vi "LEDC Control Loop 1931 Main.vi"(0 "LEDAD Port":refnum<visa-resource-name>="COM9", 1 "Enable":u8, 2 "Inten Desired":refnum<vi>, 3 "Illum Meas":refnum<vi>, 5 "Light Meter Port":refnum<visa-resource-name>="COM3", 7 "Illum Desired":dbl, 9 "Error Margin":dbl=2.0, 11 "error in (no error)":errorcluster, 12 "Illum Cal Factor":dbl=0.444212 format="%#.6f", 13 "Stop":bool) -> (4 "LEDAD Port out":refnum<visa-resource-name>, 6 "Light Meter Port out":refnum<visa-resource-name>, 8 "Illum Meas":dbl format="%#_4g", 10 "Inten Desired":dbl, 14 "Done":bool, 15 "error out":errorcluster)   [LabVIEW 2010]
panel:
  out "Flag2":bool
  out "Flag1":bool
  out "Slope":dbl format="%#_4g"
  in  "Illum 10":dbl format="%#_4g"
  out "In Progress":bool
  in  "Illum 90":dbl format="%#_4g"
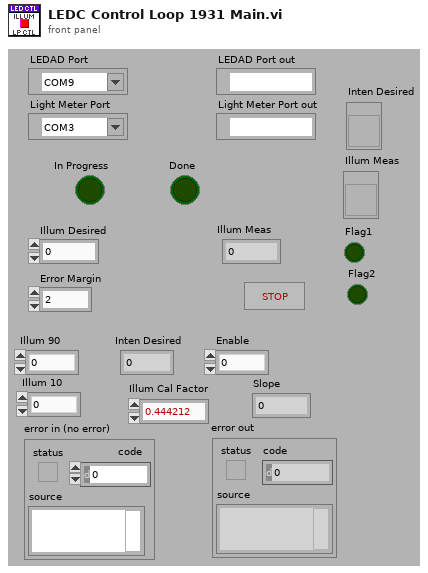
[diagram p1: front panel]
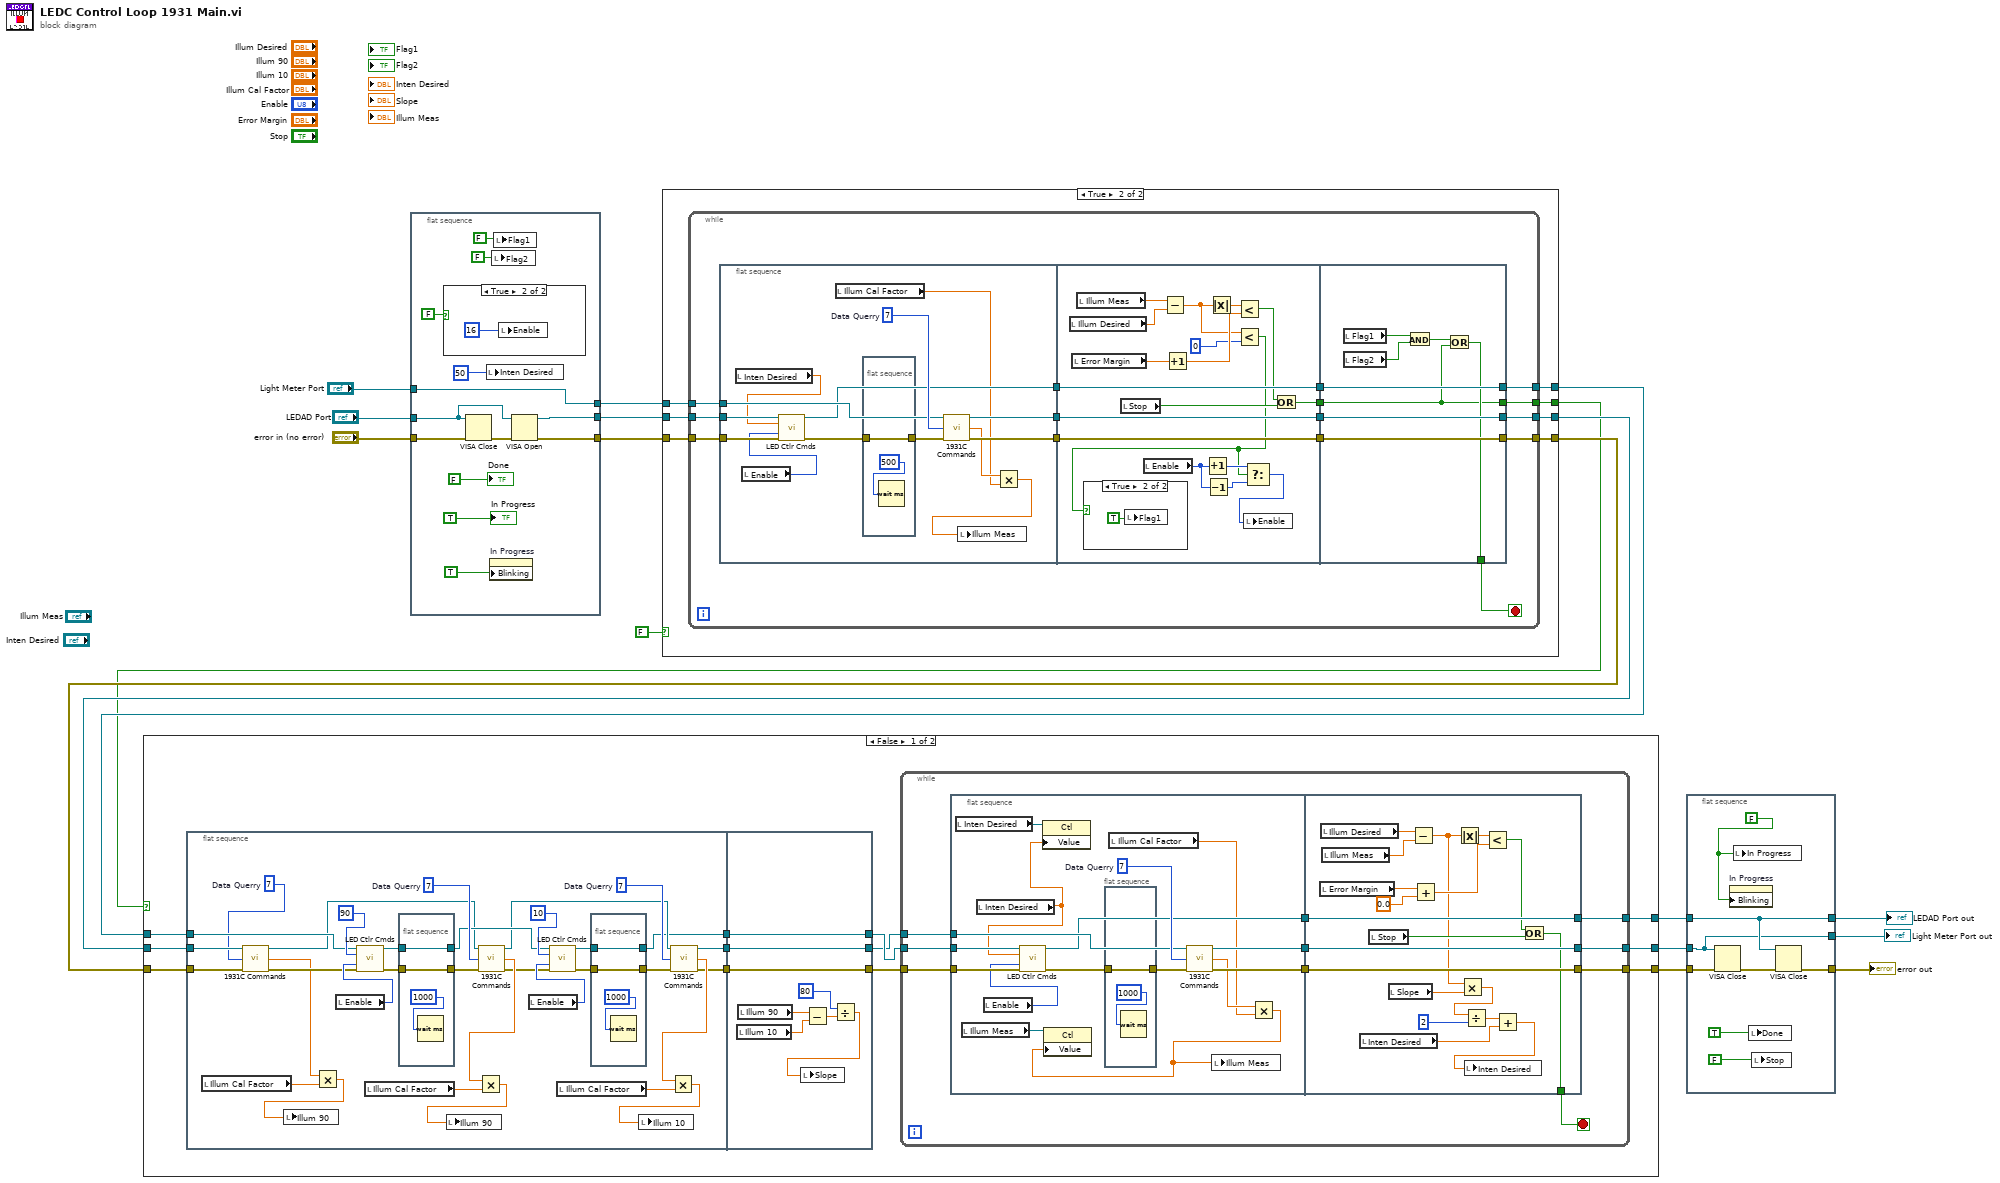
[diagram p0: block diagram]
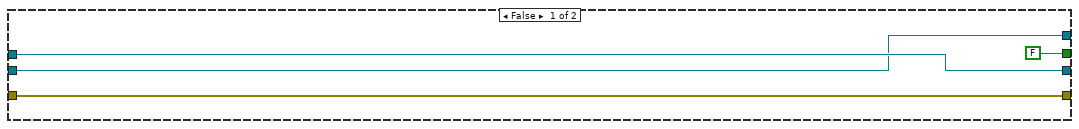
[diagram p2: hidden frame]
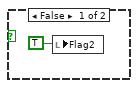
[diagram p3: hidden frame]
diagram:
  n1 = flat-sequence {
    tunnel: "LEDAD Port" -> [w23]
    tunnel: [w25] -> w14
    tunnel: "error in (no error)" -> [w26]
    tunnel: [w24] -> w16
    tunnel: "Light Meter Port" -> [w22]
    tunnel: [w22] -> w15
    frame #0 {
      n2 = case shown="True" FALSE {
        frame False {
        }
        frame True {
          n3 = local write "Enable"(16) -> ()
        }
      }
      n4 = VISA Close(VISA resource name=w23, error in (no error)=w26) -> (error out=w27:errorcluster)
      n5 = local write "Inten Desired"(50) -> ()
      n6 = property on="In Progress" class="Bool (strict)"("Blinking"=TRUE) -> ()  [unwired: 2 in, 2 out]
      n7 = local write "Flag2"(FALSE) -> ()
      n8 = local write "Flag1"(FALSE) -> ()
      n9 = VISA Open(error in (no error)=w27, VISA resource name=w23) -> (VISA resource name=w24:refnum<visa-resource-name>, error out=w25:errorcluster)  [unwired: 3 in]
      "Done" <- FALSE
      "In Progress" <- TRUE
    }
  }
  n10 = case shown="True" FALSE {
    tunnel: w16 -> [w34 w42]
    tunnel: w15 -> [w35 w41]
    tunnel: w14 -> [w33 w40]
    tunnel: [w34 w39] -> w10
    tunnel: [w35 w38] -> w9
    tunnel: [w33 w37] -> w8
    tunnel: [FALSE w36] -> w7
    frame False {
    }
    frame True {
      n11 = while {
        tunnel: w41 -> [w57]
        tunnel: w42 -> [w56]
        tunnel: w40 -> [w55]
        tunnel: [w48] -> w38
        tunnel: [w46] -> w37
        tunnel: [w47] -> w39
        tunnel: [w43] -> w36
        stop <- w44 stop-if-true
        n12 = flat-sequence {
          tunnel: w55 -> [w69]
          tunnel: w56 -> [w70]
          tunnel: w57 -> [w68]
          tunnel: [w67] -> w51
          tunnel: [w65] -> w50
          tunnel: [w66] -> w49
          tunnel: [w90] -> w54
          tunnel: [w89] -> w53
          tunnel: [w88] -> w52
          tunnel: w51 -> [w90]
          tunnel: w50 -> [w89]
          tunnel: w49 -> [w88]
          tunnel: [w75] -> w45
          tunnel: w54 -> [w101]
          tunnel: w53 -> [w100]
          tunnel: w52 -> [w99]
          tunnel: [w101] -> w48
          tunnel: [w100] -> w47
          tunnel: [w99] -> w46
          tunnel: w45 -> [w94]
          tunnel: [w95] -> w44
          tunnel: [w94] -> w43
          frame #0 {
            w71 = 7  # Data Querry
            n13 = local read "Inten Desired"() -> (w62:dbl)
            n14 = local read "Enable"() -> (w61:u8)
            n15 = call "LED Ctlr Cmds.vi"("VISA session"=w70, "Intensity"=w62, "Enable"=w61, "error in (no error)"=w69) -> ("VISA session out"=w65:refnum<visa-resource-name>, "error out"=w64:errorcluster)  [unwired: 7 in, 3 out]
            n16 = local read "Illum Cal Factor"() -> (w58:dbl)
            n17 = flat-sequence {
              tunnel: w64 -> [w73]
              tunnel: [w73] -> w63
              frame #0 {
                n18 = Wait (ms)(milliseconds to wait=500) -> ()  [unwired: 1 out]
              }
            }
            n19 = call "1931C Commands.vi"("Instrument Resource Name"=w68, "Command"=w71, "error in (no error)"=w63) -> ("VISA resource name out"=w67:refnum<visa-resource-name>, "LM Response"=w59:dbl, "error out"=w66:errorcluster)  [unwired: 8 in, 2 out]
            n20 = Multiply(x=w59, y=w58) -> (x*y=w60:dbl)
            n21 = local write "Illum Meas"(w60) -> ()
          }
          frame #1 {
            n22 = local read "Illum Desired"() -> (w85:dbl)
            n23 = local read "Error Margin"() -> (w83:dbl)
            n24 = local read "Illum Meas"() -> (w86:dbl)
            n25 = local read "Stop"() -> (w82:bool)
            n26 = local read "Enable"() -> (w77:u8)
            n27 = Subtract(x=w86, y=w85) -> (x-y=w81:dbl)
            n28 = Increment(x=w83) -> (x+1=w84:dbl)
            n29 = Increment(x=w77) -> (x+1=w78:u8)
            n30 = Decrement(x=w77) -> (x-1=w79:u8)
            n31 = Absolute Value(x=w81) -> (abs(x)=w91:dbl)
            n32 = Less?(x=w91, y=w84) -> (x < y?=w87:bool)
            n33 = Less?(x=w81, y=0) -> (x < y?=w76:bool)
            n34 = case shown="True" w76 {
              frame False {
                n35 = local write "Flag2"(TRUE) -> ()
              }
              frame True {
                n36 = local write "Flag1"(TRUE) -> ()
              }
            }
            n37 = Select(t=w78, s=w76, f=w79) -> (s? t:f=w74:u8)
            n38 = local write "Enable"(w74) -> ()
            n39 = Or(x=w87, y=w82) -> (x .or. y?=w75:bool)
          }
          frame #2 {
            n40 = local read "Flag1"() -> (w98:bool)
            n41 = local read "Flag2"() -> (w97:bool)
            n42 = And(x=w98, y=w97) -> (x .and. y?=w96:bool)
            n43 = Or(x=w96, y=w94) -> (x .or. y?=w95:bool)
          }
        }
      }
    }
  }
  n44 = case shown="False" w7 {
    tunnel: w10 -> [w105 w208]
    tunnel: w9 -> [w111 w209]
    tunnel: w8 -> [w110 w210]
    tunnel: [w106 w210] -> w6
    tunnel: [w108 w209] -> w5
    tunnel: [w107 w208] -> w4
    frame False {
      n45 = flat-sequence {
        tunnel: w111 -> [w121]
        tunnel: w110 -> [w120]
        tunnel: [w127] -> w113
        tunnel: [w126] -> w112
        tunnel: w105 -> [w125]
        tunnel: [w122] -> w104
        tunnel: [w160] -> w102
        tunnel: w113 -> [w160]
        tunnel: [w159] -> w109
        tunnel: w112 -> [w159]
        tunnel: [w155] -> w103
        tunnel: w104 -> [w155]
        frame #0 {
          w117 = 7  # Data Querry
          w134 = 7  # Data Querry
          w141 = 7  # Data Querry
          n46 = local read "Illum Cal Factor"() -> (w116:dbl)
          n47 = call "1931C Commands.vi"("Instrument Resource Name"=w121, "Command"=w117, "error in (no error)"=w120) -> ("VISA resource name out"=w119:refnum<visa-resource-name>, "LM Response"=w114:dbl, "error out"=w118:errorcluster)  [unwired: 8 in, 2 out]
          n48 = Multiply(x=w114, y=w116) -> (x*y=w115:dbl)
          n49 = local write "Illum 90"(w115) -> ()
          n50 = local read "Enable"() -> (w146:u8)
          n51 = call "LED Ctlr Cmds.vi"("VISA session"=w125, "Intensity"=90, "Enable"=w146, "error in (no error)"=w118) -> ("VISA session out"=w143:refnum<visa-resource-name>, "error out"=w144:errorcluster)  [unwired: 7 in, 3 out]
          n52 = local read "Illum Cal Factor"() -> (w138:dbl)
          n53 = flat-sequence {
            tunnel: w144 -> [w152]
            tunnel: [w152] -> w142
            tunnel: [w150] -> w124
            tunnel: w143 -> [w150]
            frame #0 {
              n54 = Wait (ms)(milliseconds to wait=1000) -> ()  [unwired: 1 out]
            }
          }
          n55 = call "1931C Commands.vi"("Instrument Resource Name"=w119, "Command"=w141, "error in (no error)"=w142) -> ("VISA resource name out"=w123:refnum<visa-resource-name>, "LM Response"=w139:dbl, "error out"=w128:errorcluster)  [unwired: 8 in, 2 out]
          n56 = Multiply(x=w139, y=w138) -> (x*y=w140:dbl)
          n57 = local write "Illum 90"(w140) -> ()
          n58 = local read "Enable"() -> (w129:u8)
          n59 = call "LED Ctlr Cmds.vi"("VISA session"=w124, "Intensity"=10, "Enable"=w129, "error in (no error)"=w128) -> ("VISA session out"=w132:refnum<visa-resource-name>, "error out"=w131:errorcluster)  [unwired: 7 in, 3 out]
          n60 = local read "Illum Cal Factor"() -> (w137:dbl)
          n61 = flat-sequence {
            tunnel: w131 -> [w149]
            tunnel: [w149] -> w133
            tunnel: [w147] -> w122
            tunnel: w132 -> [w147]
            frame #0 {
              n62 = Wait (ms)(milliseconds to wait=1000) -> ()  [unwired: 1 out]
            }
          }
          n63 = call "1931C Commands.vi"("Instrument Resource Name"=w123, "Command"=w134, "error in (no error)"=w133) -> ("VISA resource name out"=w127:refnum<visa-resource-name>, "LM Response"=w136:dbl, "error out"=w126:errorcluster)  [unwired: 8 in, 2 out]
          n64 = Multiply(x=w136, y=w137) -> (x*y=w135:dbl)
          n65 = local write "Illum 10"(w135) -> ()
        }
        frame #1 {
          n66 = local read "Illum 10"() -> (w157:dbl)
          n67 = local read "Illum 90"() -> (w158:dbl)
          n68 = Subtract(x=w158, y=w157) -> (x-y=w154:dbl)
          n69 = Divide(x=80, y=w154) -> (x/y=w156:dbl)
          n70 = local write "Slope"(w156) -> ()
        }
      }
      n71 = while {
        tunnel: w102 -> [w170]
        tunnel: w103 -> [w169]
        tunnel: w109 -> [w168]
        tunnel: [w164] -> w108
        tunnel: [w162] -> w106
        tunnel: [w163] -> w107
        stop <- w161 stop-if-true
        n72 = flat-sequence {
          tunnel: w168 -> [w184]
          tunnel: w169 -> [w185]
          tunnel: w170 -> [w183]
          tunnel: [w182] -> w167
          tunnel: [w180] -> w166
          tunnel: [w181] -> w165
          tunnel: w167 -> [w206]
          tunnel: w166 -> [w205]
          tunnel: w165 -> [w204]
          tunnel: [w191] -> w161
          tunnel: [w206] -> w164
          tunnel: [w205] -> w163
          tunnel: [w204] -> w162
          frame #0 {
            w186 = 7  # Data Querry
            n73 = local read "Inten Desired"() -> (w174:refnum<vi>)
            n74 = local read "Illum Meas"() -> (w172:refnum<vi>)
            n75 = local read "Inten Desired"() -> (w173:dbl)
            n76 = local read "Enable"() -> (w177:u8)
            n77 = call "LED Ctlr Cmds.vi"("VISA session"=w185, "Intensity"=w173, "Enable"=w177, "error in (no error)"=w184) -> ("VISA session out"=w180:refnum<visa-resource-name>, "error out"=w179:errorcluster)  [unwired: 7 in, 3 out]
            n78 = property class="Ctl"(reference=w174, "Value"=w173) -> ()  [unwired: 1 in, 2 out]
            n79 = flat-sequence {
              tunnel: w179 -> [w188]
              tunnel: [w188] -> w178
              frame #0 {
                n80 = Wait (ms)(milliseconds to wait=1000) -> ()  [unwired: 1 out]
              }
            }
            n81 = local read "Illum Cal Factor"() -> (w175:dbl)
            n82 = call "1931C Commands.vi"("Instrument Resource Name"=w183, "Command"=w186, "error in (no error)"=w178) -> ("VISA resource name out"=w182:refnum<visa-resource-name>, "LM Response"=w176:dbl, "error out"=w181:errorcluster)  [unwired: 8 in, 2 out]
            n83 = Multiply(x=w176, y=w175) -> (x*y=w171:dbl)
            n84 = property class="Ctl"(reference=w172, "Value"=w171) -> ()  [unwired: 1 in, 2 out]
            n85 = local write "Illum Meas"(w171) -> ()
          }
          frame #1 {
            n86 = local read "Error Margin"() -> (w190:dbl)
            n87 = local read "Illum Desired"() -> (w202:dbl)
            n88 = local read "Illum Meas"() -> (w201:dbl)
            n89 = local read "Inten Desired"() -> (w193:dbl)
            n90 = local read "Stop"() -> (w199:bool)
            n91 = local read "Slope"() -> (w197:dbl)
            n92 = Subtract(x=w202, y=w201) -> (x-y=w195:dbl)
            n93 = Add(x=w190, y=0.0) -> (x+y=w200:dbl)
            n94 = Absolute Value(x=w195) -> (abs(x)=w207:dbl)
            n95 = Multiply(x=w195, y=w197) -> (x*y=w194:dbl)
            n96 = Divide(x=w194, y=2) -> (x/y=w196:dbl)
            n97 = Less?(x=w207, y=w200) -> (x < y?=w203:bool)
            n98 = Add(x=w196, y=w193) -> (x+y=w192:dbl)
            n99 = local write "Inten Desired"(w192) -> ()
            n100 = Or(x=w203, y=w199) -> (x .or. y?=w191:bool)
          }
        }
      }
    }
    frame True {
    }
  }
  n101 = flat-sequence {
    tunnel: w5 -> [w214]
    tunnel: w6 -> [w216]
    tunnel: [w215] -> w2
    tunnel: w4 -> [w215]
    tunnel: [w214] -> w3
    tunnel: [w212] -> w17
    frame #0 {
      w218 = FALSE
      n102 = VISA Close(VISA resource name=w214, error in (no error)=w216) -> (error out=w213:errorcluster)
      n103 = property on="In Progress" class="Bool (strict)"("Blinking"=w218) -> ()  [unwired: 2 in, 2 out]
      n104 = local write "In Progress"(w218) -> ()
      n105 = local write "Done"(TRUE) -> ()
      n106 = local write "Stop"(FALSE) -> ()
      n107 = VISA Close(VISA resource name=w215, error in (no error)=w213) -> (error out=w212:errorcluster)
    }
  }
  "error out" <- w17
  "Light Meter Port out" <- w3
  "LEDAD Port out" <- w2
